vi "EminemBegin.vi"(6 "error in (no error)":errorcluster) -> (0 "error out":errorcluster)   [LabVIEW 2023]
doc: "Opens motors and sensors for Eminem subassembly\nInputs:\n--Error in--error type\nOutputs:\n--Error out--error type"
uses:
  <vilib>/Rock Robotics/WPI/ThirdParty/REV Robotics/REVLib/Typedef/Spark MAX Idle Mode.ctl
  <vilib>/Rock Robotics/WPI/ThirdParty/REV Robotics/REVLib/Typedef/Spark MAX Motor Type.ctl
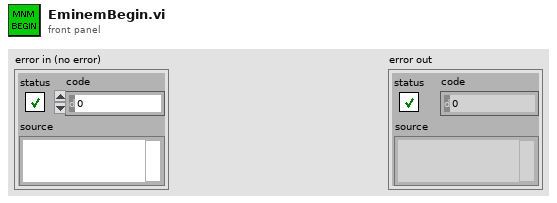
[diagram p1: front panel]
types:
  T1 = typedef "Spark MAX Idle Mode.ctl" = enum16{"Coast", "Brake"}
  T2 = typedef "Spark MAX Motor Type.ctl" = enum16{"Brushed", "Brushless"}
  T3 = typedef "WPI_MotorControlDeviceRef.ctl" = cluster{"DeviceStatus":errorcluster, "Type":T4, "PWM":cluster{"PWM Channel":T5, "DeadBand":T6}, "CAN":cluster{"Device Number":u8, "SetOutput VI Ref":variant, "GetOutput VI Ref":variant, "Enable VI Ref":variant, "Disable VI Ref":variant, "Data":variant}, "Invert":bool, "DIO PWM":cluster{"PWM \"Enable\" Channel":T5, "DIOChannel":T7, "PWM Rate":dbl}}
  T4 = typedef "WPI_MotorControlType.ctl" = enum16{"PWM", "CAN", "DIO PWM"}
  T5 = typedef "FPGA_DIOPWMChannel.ctl" = enum8{"PWM 0", "PWM 1", "PWM 2", "PWM 3", "PWM 4", "PWM 5", "PWM 6", "PWM 7", "PWM 8", "PWM 9", "PWM MXP 0", "PWM MXP 1", "PWM MXP 2", "PWM MXP 3", "PWM MXP 4", "PWM MXP 5", "PWM MXP 6", "PWM MXP 7", "PWM MXP 8", "PWM MXP 9", "Invalid"}
  T6 = typedef "WPI_PWMDeadband.ctl" = cluster{"Name":string, "maxPositivePwm":i32, "minPositivePwm":i32, "centerPwm":i32, "maxNegativePwm":i32, "minNegativePwm":i32, "angularRange":u16}
  T7 = typedef "FPGA_DIOChannel.ctl" = enum8{"DIO 0", "DIO 1", "DIO 2", "DIO 3", "DIO 4", "DIO 5", "DIO 6", "DIO 7", "DIO 8", "DIO 9", "DIO MXP 0", "DIO MXP 1", "DIO MXP 2", "DIO MXP 3", "DIO MXP 4", "DIO MXP 5", "DIO MXP 6", "DIO MXP 7", "DIO MXP 8", "DIO MXP 9", "DIO MXP 10", "DIO MXP 11", "DIO MXP 12", "DIO MXP 13", "DIO MXP 14", "DIO MXP 15", "SPI Port CS1", "SPI Port CS2", "SPI Port CS3", "SPI Port MISO", "SPI Port MOSI", "Invalid"}
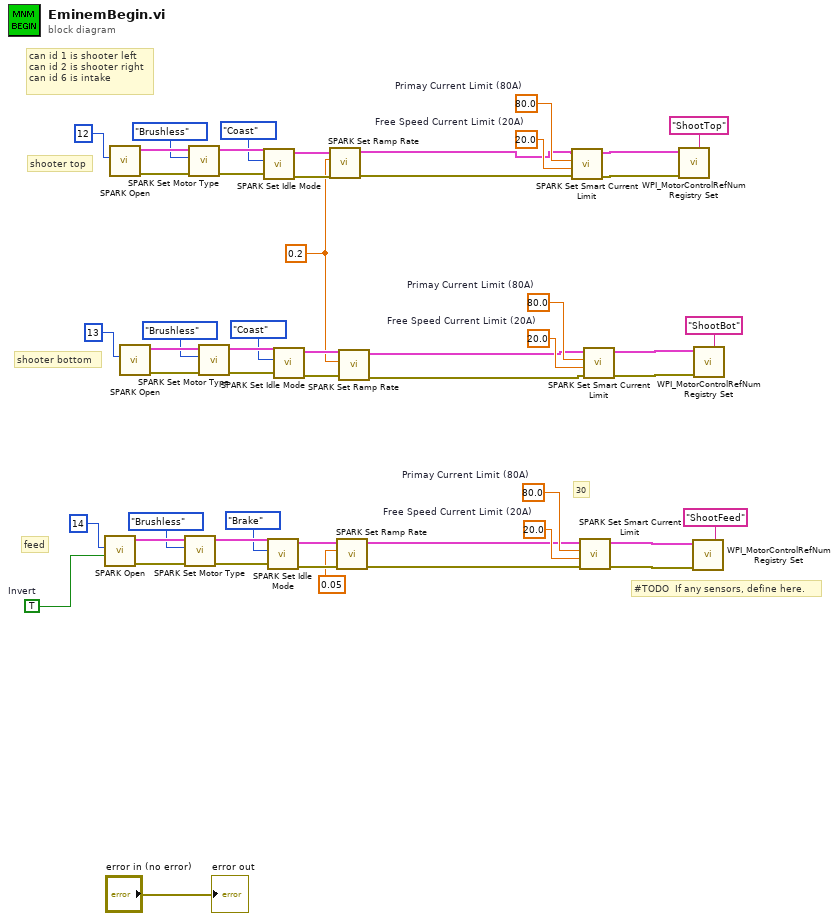
[diagram p0: block diagram]
diagram:
  w1 = TRUE  # Invert
  w8 = 20.0  # Free Speed Current Limit (20A)
  w9 = 80.0  # Primay Current Limit (80A)
  w14 = 20.0  # Free Speed Current Limit (20A)
  w15 = 80.0  # Primay Current Limit (80A)
  w16 = 20.0  # Free Speed Current Limit (20A)
  w17 = 80.0  # Primay Current Limit (80A)
  w21 = 0.2
  # "30"
  # "#TODO  If any sensors, define here."
  # "feed"
  # "shooter bottom"
  # "shooter top"
  # "can id 1 is shooter left\ncan id 2 is shooter right\ncan id 6 is intake"
  n1 = call <vilib>:"SPARK Open.vi"("Invert"=w1, "Device Number"=14) -> ("error out"=w31:errorcluster, "MotorControlDeviceRef"=w33:T3)  [unwired: 8 in]
  n2 = call <vilib>:"SPARK Open.vi"("Device Number"=12) -> ("error out"=w47:errorcluster, "MotorControlDeviceRef"=w49:T3)  [unwired: 9 in]
  n3 = call <vilib>:"SPARK Open.vi"("Device Number"=13) -> ("error out"=w39:errorcluster, "MotorControlDeviceRef"=w41:T3)  [unwired: 9 in]
  n4 = call <vilib>:"SPARK Set Motor Type.vi"("error in (no error)"=w31, "Motor Type"=Spark_MAX_Motor_Type."Brushless", "MotorControlDevRef"=w33) -> ("error out"=w30:errorcluster, "MotorControlDeviceRef"=w32:T3)  [unwired: 7 in]
  n5 = call <vilib>:"SPARK Set Motor Type.vi"("error in (no error)"=w47, "Motor Type"=Spark_MAX_Motor_Type."Brushless", "MotorControlDevRef"=w49) -> ("error out"=w46:errorcluster, "MotorControlDeviceRef"=w48:T3)  [unwired: 7 in]
  n6 = call <vilib>:"SPARK Set Motor Type.vi"("error in (no error)"=w39, "Motor Type"=Spark_MAX_Motor_Type."Brushless", "MotorControlDevRef"=w41) -> ("error out"=w38:errorcluster, "MotorControlDeviceRef"=w40:T3)  [unwired: 7 in]
  n7 = call <vilib>:"SPARK Set Idle Mode.vi"("error in (no error)"=w46, "Idle Mode"=Spark_MAX_Idle_Mode."Coast", "MotorControlDeviceRef in"=w48) -> ("error out"=w25:errorcluster, "MotorControlDeviceRef out"=w24:T3)  [unwired: 7 in]
  n8 = call <vilib>:"SPARK Set Idle Mode.vi"("error in (no error)"=w30, "Idle Mode"=Spark_MAX_Idle_Mode."Brake", "MotorControlDeviceRef in"=w32) -> ("error out"=w22:errorcluster, "MotorControlDeviceRef out"=w23:T3)  [unwired: 7 in]
  n9 = call <vilib>:"SPARK Set Idle Mode.vi"("error in (no error)"=w38, "Idle Mode"=Spark_MAX_Idle_Mode."Coast", "MotorControlDeviceRef in"=w40) -> ("error out"=w26:errorcluster, "MotorControlDeviceRef out"=w27:T3)  [unwired: 7 in]
  n10 = call <vilib>:"SPARK Set Ramp Rate.vi"("error in (no error)"=w25, "Seconds from neutral to full (0)"=w21, "MotorControlDeviceRef in"=w24) -> ("error out"=w6:errorcluster, "MotorControlDeviceRef"=w7:T3)  [unwired: 7 in]
  n11 = call <vilib>:"SPARK Set Ramp Rate.vi"("error in (no error)"=w22, "Seconds from neutral to full (0)"=0.05, "MotorControlDeviceRef in"=w23) -> ("error out"=w3:errorcluster, "MotorControlDeviceRef"=w2:T3)  [unwired: 7 in]
  n12 = call <vilib>:"SPARK Set Ramp Rate.vi"("error in (no error)"=w26, "Seconds from neutral to full (0)"=w21, "MotorControlDeviceRef in"=w27) -> ("error out"=w12:errorcluster, "MotorControlDeviceRef"=w13:T3)  [unwired: 7 in]
  n13 = call <vilib>:"SPARK Set Smart Current Limit.vi"("error in (no error)"=w6, "Free Speed Current Limit (20A)"=w8, "Primay Current Limit (80A)"=w9, "MotorControlDeviceRef in"=w7) -> ("error out"=w4:errorcluster, "MotorControlDeviceRef out"=w5:T3)  [unwired: 6 in]
  n14 = call <vilib>:"SPARK Set Smart Current Limit.vi"("error in (no error)"=w3, "Free Speed Current Limit (20A)"=w16, "Primay Current Limit (80A)"=w17, "MotorControlDeviceRef in"=w2) -> ("error out"=w18:errorcluster, "MotorControlDeviceRef out"=w19:T3)  [unwired: 6 in]
  n15 = call <vilib>:"SPARK Set Smart Current Limit.vi"("error in (no error)"=w12, "Free Speed Current Limit (20A)"=w14, "Primay Current Limit (80A)"=w15, "MotorControlDeviceRef in"=w13) -> ("error out"=w10:errorcluster, "MotorControlDeviceRef out"=w11:T3)  [unwired: 6 in]
  n16 = call <vilib>:"WPI_MotorControlRefNum Registry Set.vi"("error in (no error)"=w4, "refnum name"="ShootTop", "MotorControlDevRef"=w5) -> ()  [unwired: 7 in, 2 out]
  n17 = call <vilib>:"WPI_MotorControlRefNum Registry Set.vi"("error in (no error)"=w18, "refnum name"="ShootFeed", "MotorControlDevRef"=w19) -> ()  [unwired: 7 in, 2 out]
  n18 = call <vilib>:"WPI_MotorControlRefNum Registry Set.vi"("error in (no error)"=w10, "refnum name"="ShootBot", "MotorControlDevRef"=w11) -> ()  [unwired: 7 in, 2 out]
  "error out" <- "error in (no error)"
